vi "sendRGBimg.vi"() -> ()   [LabVIEW 2018, in "LV-Julia_ZMQ-Roundtrip_lib.lvlib"]
uses:
  LV-Julia_ZMQ-Roundtrip_lib.lvlib
  example args cluster.ctl
  detailed error info.ctl
  StackFrame.ctl
  example server response cluster.ctl
  Server or client state.ctl
  Commands v2.ctl
  commands LV2Jl.ctl
  Julia functions enum.ctl
  5d385633-7562-4640-8300-e9530f023818.vi
  c1ad7611-f00e-47ba-b950-502655f00f75.vi
  56e59d91-b000-48d4-98d3-11fae75f7a72.vi
  131ce374-9601-4316-a426-5169ad24f463.vi
  c49a53f7-dacd-4aad-9c2e-667c4b60ae7c.vi
  cb7a600e-1a3f-45a0-9149-1773accb9ab7.vi
  5d385633-7562-4640-8300-e9530f023818.vi/39034429-44f1-49eb-8b93-01b3577d4bbb.vi
  c1ad7611-f00e-47ba-b950-502655f00f75.vi/c20b7bce-7184-44ac-a221-24bd74e8a069.vi
  c1ad7611-f00e-47ba-b950-502655f00f75.vi/b679c96a-12bc-4fd8-b1fa-0e060ec68c49.vi
  c1ad7611-f00e-47ba-b950-502655f00f75.vi/0532bd6e-2df5-4c62-b78f-3fbcd680d2d7.vi
  56e59d91-b000-48d4-98d3-11fae75f7a72.vi/afa31c40-cfad-4424-8ad1-0d826b484572.vi
  56e59d91-b000-48d4-98d3-11fae75f7a72.vi/5df44c0f-7a44-4987-b105-2b8f6222c511.vi
  56e59d91-b000-48d4-98d3-11fae75f7a72.vi/a7c2328a-2d06-4c0e-8cd3-214f0a2bf022.vi
  131ce374-9601-4316-a426-5169ad24f463.vi/a827da90-2120-4d2c-9db5-3fec82af9c5d.vi
  131ce374-9601-4316-a426-5169ad24f463.vi/028239c2-02b4-461b-80d8-33e46285812d.vi
  131ce374-9601-4316-a426-5169ad24f463.vi/8b056bee-da33-4f9d-affb-232afdb11d3e.vi
  c49a53f7-dacd-4aad-9c2e-667c4b60ae7c.vi/86660411-e67f-4121-95dc-5e42147ac36e.vi
  c49a53f7-dacd-4aad-9c2e-667c4b60ae7c.vi/08ba786e-4a78-441a-9161-a5b743b68032.vi
  c49a53f7-dacd-4aad-9c2e-667c4b60ae7c.vi/61ee4b15-9c18-4f14-9227-04bb8a8aef80.vi
  5d385633-7562-4640-8300-e9530f023818.vi/39034429-44f1-49eb-8b93-01b3577d4bbb.vi/c666953e-88d8-4c63-ac9c-57e5f8a328dd.vi
  check ID validity.vi
  <vilib>/Utility/error.llb/Error Cluster From Error Code.vi
  convert Jl functions enum to string.vi
  bindata_descr to JSON.vi
  check cluster field names.vi
  concat JSON.vi
panel:
  out "new picture":picture
  out "parsed response 2":cluster{"elem":dbl}
  out "binary data":u8[](array[numeric])
  in  "separate arg2":cluster{"arg2":dbl}={"arg2"=2.14}
  in  "separate arg 1":cluster{"arg1":i32}={"arg1"=2}
  in  "index to return":cluster{"idx":u16[]}={"idx"=[1, 1, 1]} {"idx" min=1}
  in  "stop LV only":bool
  out "JSON args":string
  out "LV Client state out":T1
  out "Jl Server state out":T1
  out "size(s)":i32
  out "unsigned byte array":u8[](array[numeric])
  out "short err code":u8
  in  "go once":bool
  out "JSON received":string
  out "parsed response":T2 {"bin_lng" format="%.0e"}
  out "final error":errorcluster
  out "current error":errorcluster
  out "status":T3
  in  "stop":bool
  in  "joint args":T5={"arg1"=1, "arg2"=3.14}
  # "(myf2)"
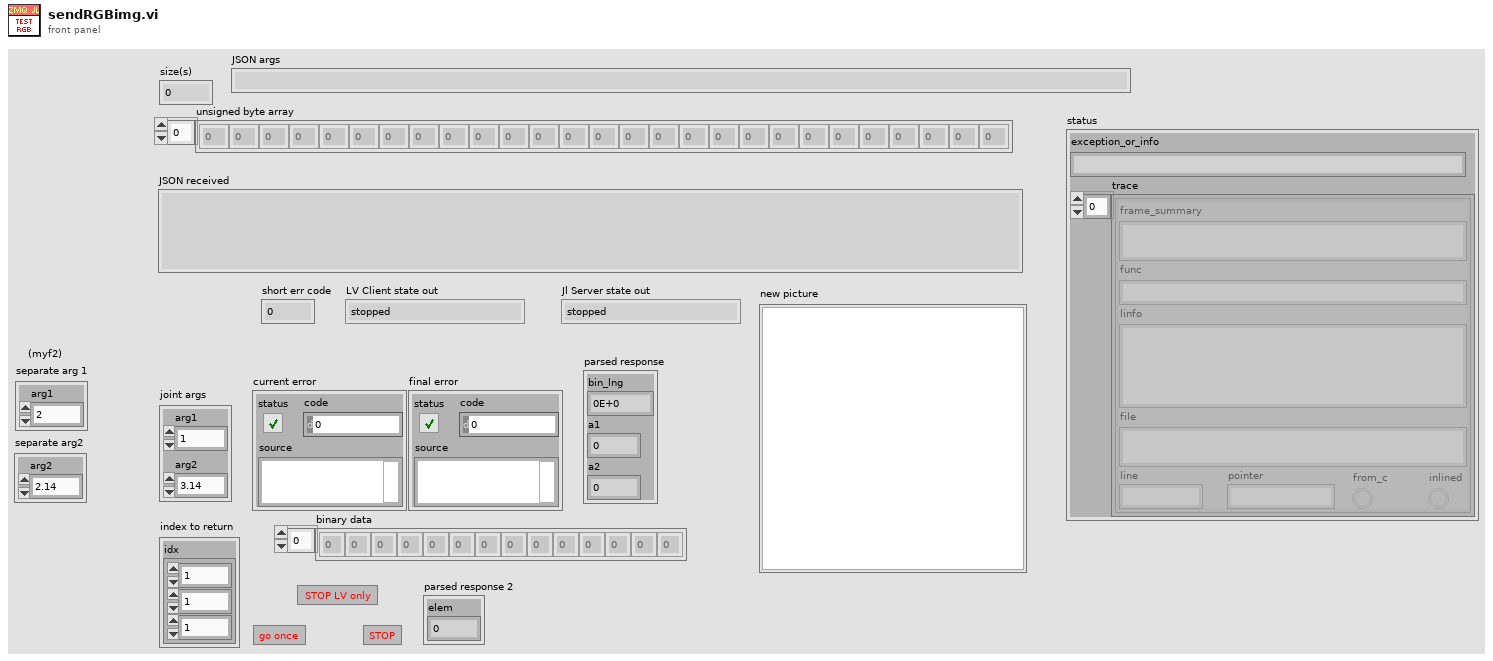
[diagram p1: front panel]
types:
  T1 = typedef "LV-Julia_ZMQ-Roundtrip_lib.lvlib/Server or client state.ctl" = enum16{"stopped", "running", "unknown"}
  T2 = typedef "example server response cluster.ctl" = cluster{"bin_lng":i32, "a1":i32, "a2":dbl}
  T3 = typedef "LV-Julia_ZMQ-Roundtrip_lib.lvlib/detailed error info.ctl" = cluster{"exception_or_info":string, "trace":T4[]}
  T4 = typedef "LV-Julia_ZMQ-Roundtrip_lib.lvlib/StackFrame.ctl" = cluster{"frame_summary":string, "func":string, "linfo":string, "file":string, "line":i32, "pointer":u64, "from_c":bool, "inlined":bool}
  T5 = typedef "example args cluster.ctl" = cluster{"arg1":i32, "arg2":dbl}
  T6 = typedef "LV-Julia_ZMQ-Roundtrip_lib.lvlib/Commands v2.ctl" = enum16{"Start Jl-server & Init LV-client", "Send request & Get response ", "Stop Jl-server & Cleanup LV-client", "Cleanup LV-client", "Start Jl-server", "Stop Jl-server", "Init LV-Client", "Cleanup LV-Client", "(not allowed)", "Set LV Client state", "Set Jl Server state"}
  T7 = typedef "LV-Julia_ZMQ-Roundtrip_lib.lvlib/Julia functions enum.ctl" = enum16{"myf1", "myf2", "myf3", "test_bin2nums", "test_rgbimg", "numarr_loopback", "numarrs_lpbk", "Not_a_Fun"}
  T8 = typedef "commands LV2Jl.ctl" = u8
  T9 = typedef "imagedata.ctl" = cluster{"image type":i32, "image depth":i32, "image":u8[], "mask":u8[], "colors":u32[], "Rectangle":cluster{"left":i16, "top":i16, "right":i16, "bottom":i16}}
  T10 = typedef "Bindata&description.ctl" = cluster{"bindata_descr":T11[], "bindata":u8[]}
  T11 = typedef "LV-Julia_ZMQ-Roundtrip_lib.lvlib/Bindata description.ctl" = cluster{"nofbytes":i32, "numtype":string, "start":i32, "arrdims":i32[], "kwarg_name":string, "category":string}
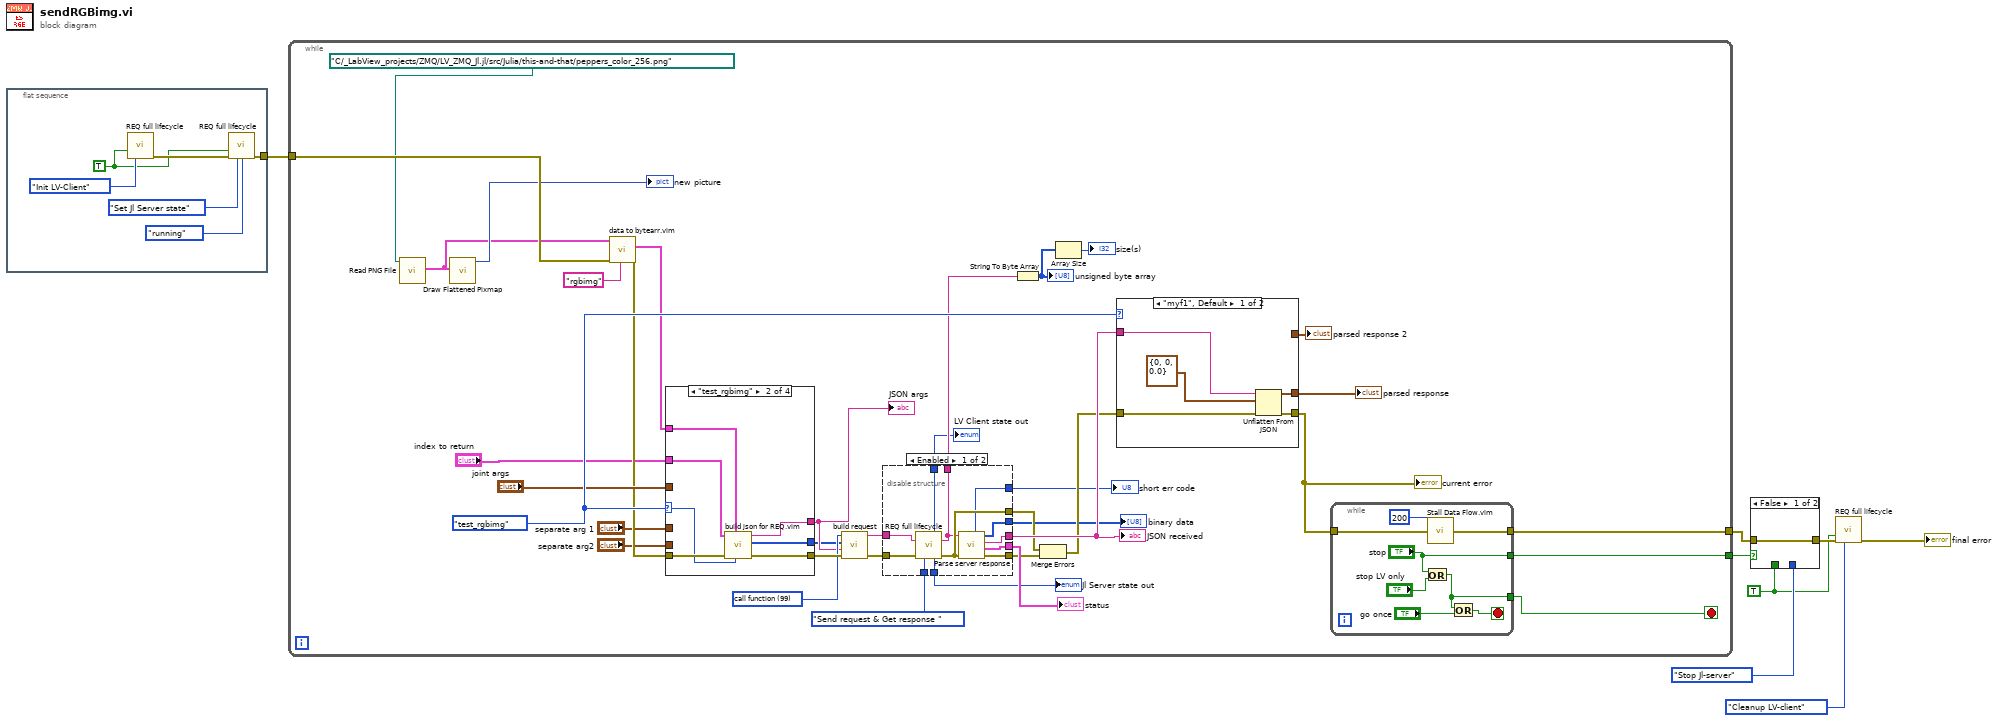
[diagram p0: block diagram]
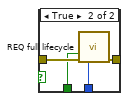
[diagram p2: hidden frame]
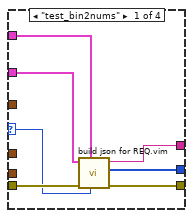
[diagram p4: hidden frame]
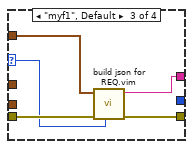
[diagram p5: hidden frame]
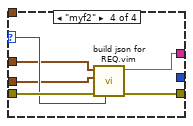
[diagram p6: hidden frame]
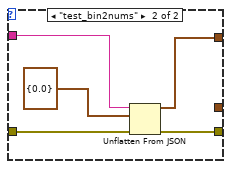
[diagram p7: hidden frame]
diagram:
  w3 = TRUE ("Force command")
  n1 = flat-sequence {
    tunnel: [w12] -> w2
    frame #0 {
      w10 = TRUE ("Force command")
      n2 = call "REQ full lifecycle.vi"("Force command"=w10, "command"=Commands_v2."Init LV-Client") -> ("error out"=w13:errorcluster)  [unwired: 10 in, 3 out]
      n3 = call "REQ full lifecycle.vi"("Force command"=w10, "error in"=w13, "command"=Commands_v2."Set Jl Server state", "Jl Server state in"=Server_or_client_state."running") -> ("error out"=w12:errorcluster)  [unwired: 8 in, 3 out]
    }
  }
  n4 = while {
    tunnel: w2 -> [w26]
    tunnel: [w41] -> w8
    tunnel: [w25] -> w1
    stop <- w40 stop-if-true
    w37 = Julia_functions_enum."test_rgbimg" ("fun2call")
    w38 = T8 99 items=["call function"=99, "ping"=112, "stop"=115] ("Command")
    n5 = call <vilib>:"Read PNG File.vi"("path to PNG file"=path "C:/_LabView_projects/ZMQ/LV_ZMQ_Jl.jl/src/Julia/this-and-that/peppers_color_256.png" ("Path")) -> ("image data"=w15:T9)  [unwired: 8 in, 2 out]
    n6 = call <vilib>:"Draw Flattened Pixmap.vi"("image data"=w15) -> ("new picture"=→"new picture":picture)  [unwired: 8 in]
    n7 = call "data to bytearr.vim"("kwarg_name"="rgbimg" ("Tag"), "error in (no error)"=w26, "data in"=w15) -> ("error out"=w35:errorcluster, "Bindata & descr out"=w34:T10)  [unwired: 6 in, 1 out]
    n8 = case shown="\"test_rgbimg\"" w37 {
      selector: w37 -> [w66 w73 w78 w85]
      tunnel: [w69 w76 w81 w87] -> w48
      tunnel: [w68 w75 w80 w86] -> w24
      tunnel: w35 -> [w70 w77 w82 w88]
      tunnel: w34 -> [w64 w71 _ _]
      tunnel: "joint args" -> [_ _ w79 _]
      tunnel: "index to return" -> [w67 w74 _ _]
      tunnel: [w65 w72 _ _] -> w22
      tunnel: "separate arg 1" -> [_ _ _ w84]
      tunnel: "separate arg2" -> [_ _ _ w83]
      frame "test_bin2nums" {
        n9 = call "build json for REQ.vim"("fun2call"=w66, "Bindata & descr in"=w64, "error in (no error)"=w70, "Arguments 1"=w67) -> ("error out"=w69:errorcluster, "bindata out"=w65:u8[], "JSON string out"=w68:string)  [unwired: 5 in]
      }
      frame "test_rgbimg" {
        n10 = call "build json for REQ.vim"("fun2call"=w73, "Bindata & descr in"=w71, "error in (no error)"=w77, "Arguments 1"=w74) -> ("error out"=w76:errorcluster, "bindata out"=w72:u8[], "JSON string out"=w75:string)  [unwired: 5 in]
      }
      frame "myf1", Default {
        n11 = call "build json for REQ.vim"("fun2call"=w78, "error in (no error)"=w82, "Arguments 1"=w79) -> ("error out"=w81:errorcluster, "JSON string out"=w80:string)  [unwired: 6 in, 1 out]
      }
      frame "myf2" {
        n12 = call "build json for REQ.vim"("fun2call"=w85, "error in (no error)"=w88, "Arguments 2"=w83, "Arguments 1"=w84) -> ("error out"=w87:errorcluster, "JSON string out"=w86:string)  [unwired: 5 in, 1 out]
      }
    }
    "JSON args" <- w24
    n13 = call "build request.vi"("error in (no error)"=w48, "JSON data"=w24, "binary data"=w22, "Command"=w38) -> ("error out"=w46:errorcluster, "REQ string"=w47:string)  [unwired: 6 in]
    n14 = disable-structure shown="Enabled" {
      disable-tunnel: [w63 _] -> w51
      disable-tunnel: [w62 _] -> w50
      disable-tunnel: w47 -> [w61 _]
      disable-tunnel: w46 -> [w60 _]
      disable-tunnel: [w59 _] -> w45
      disable-tunnel: [w58 _] -> w44
      disable-tunnel: Commands_v2."Send request & Get response " ("command") -> [w57 _]
      disable-tunnel: [w56 _] -> w32
      disable-tunnel: [w55 _] -> w31
      disable-tunnel: [w54 _] -> w28
      disable-tunnel: [w53 _] -> w27
      disable-tunnel: [w52 _] -> w19
      frame Enabled {
        n15 = call "REQ full lifecycle.vi"("data to send"=w61, "error in"=w60, "command"=w57) -> ("LV Client state out"=w53:T1, "server response"=w55:string, "Jl Server state out"=w54:T1, "error out"=w58:errorcluster)  [unwired: 9 in]
        n16 = call "Parse server response.vi"("error in (no error)"=w58, "server response in"=w55) -> ("error out"=w59:errorcluster, "detailed error info"=w63:T3, "JSON out"=w62:string, "binary data"=w52:u8[], "return code"=w56:u8)  [unwired: 3 in, 2 out]
      }
      frame Disabled {
      }
    }
    "status" <- w51
    "JSON received" <- w50
    "short err code" <- w32
    "Jl Server state out" <- w28
    "LV Client state out" <- w27
    "binary data" <- w19
    n17 = String To Byte Array(string=w31) -> (unsigned byte array=w30:u8[])
    "unsigned byte array" <- w30
    n18 = Merge Errors(w44, w45) -> (w49:errorcluster)
    n19 = Array Size(array=w30) -> (size(s)=→"size(s)":i32)
    n20 = case shown="\"myf1\", Default" w37 {
      tunnel: w50 -> [w101 w106]
      tunnel: w49 -> [w100 w105]
      tunnel: [w99 w104] -> w42
      tunnel: [w98 _] -> w39
      tunnel: [_ w102] -> w18
      frame "myf1", Default {
        n21 = Unflatten From JSON(JSON string=w101, type and defaults=T2 {"bin_lng"=0, "a1"=0, "a2"=0.0} ("parsed response"), error in (no error)=w100) -> (value=w98:T2, error out=w99:errorcluster)  [unwired: 4 in]
      }
      frame "test_bin2nums" {
        n22 = Unflatten From JSON(JSON string=w106, type and defaults=cluster{"elem":dbl} {"elem"=0.0} ("parsed response"), error in (no error)=w105) -> (value=w102:cluster{"elem":dbl}, error out=w104:errorcluster)  [unwired: 4 in]
      }
    }
    "current error" <- w42
    "parsed response" <- w39
    "parsed response 2" <- w18
    n23 = while {
      tunnel: w42 -> [w96]
      tunnel: [w95] -> w41
      tunnel: [w91] -> w40
      tunnel: ["stop"] -> w25
      stop <- w92 stop-if-true
      n24 = Or(x="stop", y="stop LV only") -> (x .or. y?=w91:bool)
      n25 = call "Stall Data Flow.vim"("value in"=w96, "milliseconds to wait"=u32 200) -> ("value out"=w95:errorcluster)  [unwired: 1 out]
      n26 = Or(x=w91, y="go once") -> (x .or. y?=w92:bool)
    }
  }
  n27 = case shown="False" w1 {
    tunnel: w8 -> [w107 w111]
    tunnel: Commands_v2."Stop Jl-server" ("command") -> [_ w110]
    tunnel: [w107 w109] -> w6
    tunnel: w3 -> [_ w108]
    frame False {
    }
    frame True {
      n28 = call "REQ full lifecycle.vi"("Force command"=w108, "error in"=w111, "command"=w110) -> ("error out"=w109:errorcluster)  [unwired: 9 in, 3 out]
    }
  }
  n29 = call "REQ full lifecycle.vi"("Force command"=w3, "error in"=w6, "command"=Commands_v2."Cleanup LV-client") -> ("error out"=→"final error":errorcluster)  [unwired: 9 in, 3 out]
